vi "Reacquire Image.vi"(6 "Console Log in":refnum<class "Console Log.lvclass">, 7 "Gantry in":refnum<class "Gantry Class.lvclass">, 8 "error in":errorcluster, 9 "Tool Chuck?":T1(ring), 10 "Chuck":i32, 11 "Fiducial Image In":T3) -> (0 "error out":errorcluster, 3 "Fiducial Image Out":T3, 4 "Console Log out":refnum<class "Console Log.lvclass">, 5 "Gantry out":refnum<class "Gantry Class.lvclass">)   [LabVIEW 2011]
uses:
  Shared Components/Utils/Type Definitions/Fiducial Image.ctl
  Shared Components/Vec3d Class/Vec3d Class.lvclass
  Shared Components/Utils/Type Definitions/Physical Image.ctl
  <vilib>/vision/Image Controls.llb/IMAQ Image.ctl
  Shared Components/Utils/Type Definitions/Fiducial with Source.ctl
  Shared Components/Gantry Class/Gantry Class.lvclass
  Console Log/Console Log.lvclass
  Shared Components/Config Manager Class/Type Definitions/Named Position.ctl
  Shared Components/Config Manager Class/Type Definitions/Camera Enum.ctl
panel:
  out "Current Position":cluster{"X":dbl, "Y":dbl, "Z":dbl}
  in  "Accept":bool
  out "Preview":T2(plugin-control)
  # "Use MPG To locate fiducial\nand bring it into focus.\n\nClick \"Accept\" when\nsatisfied."
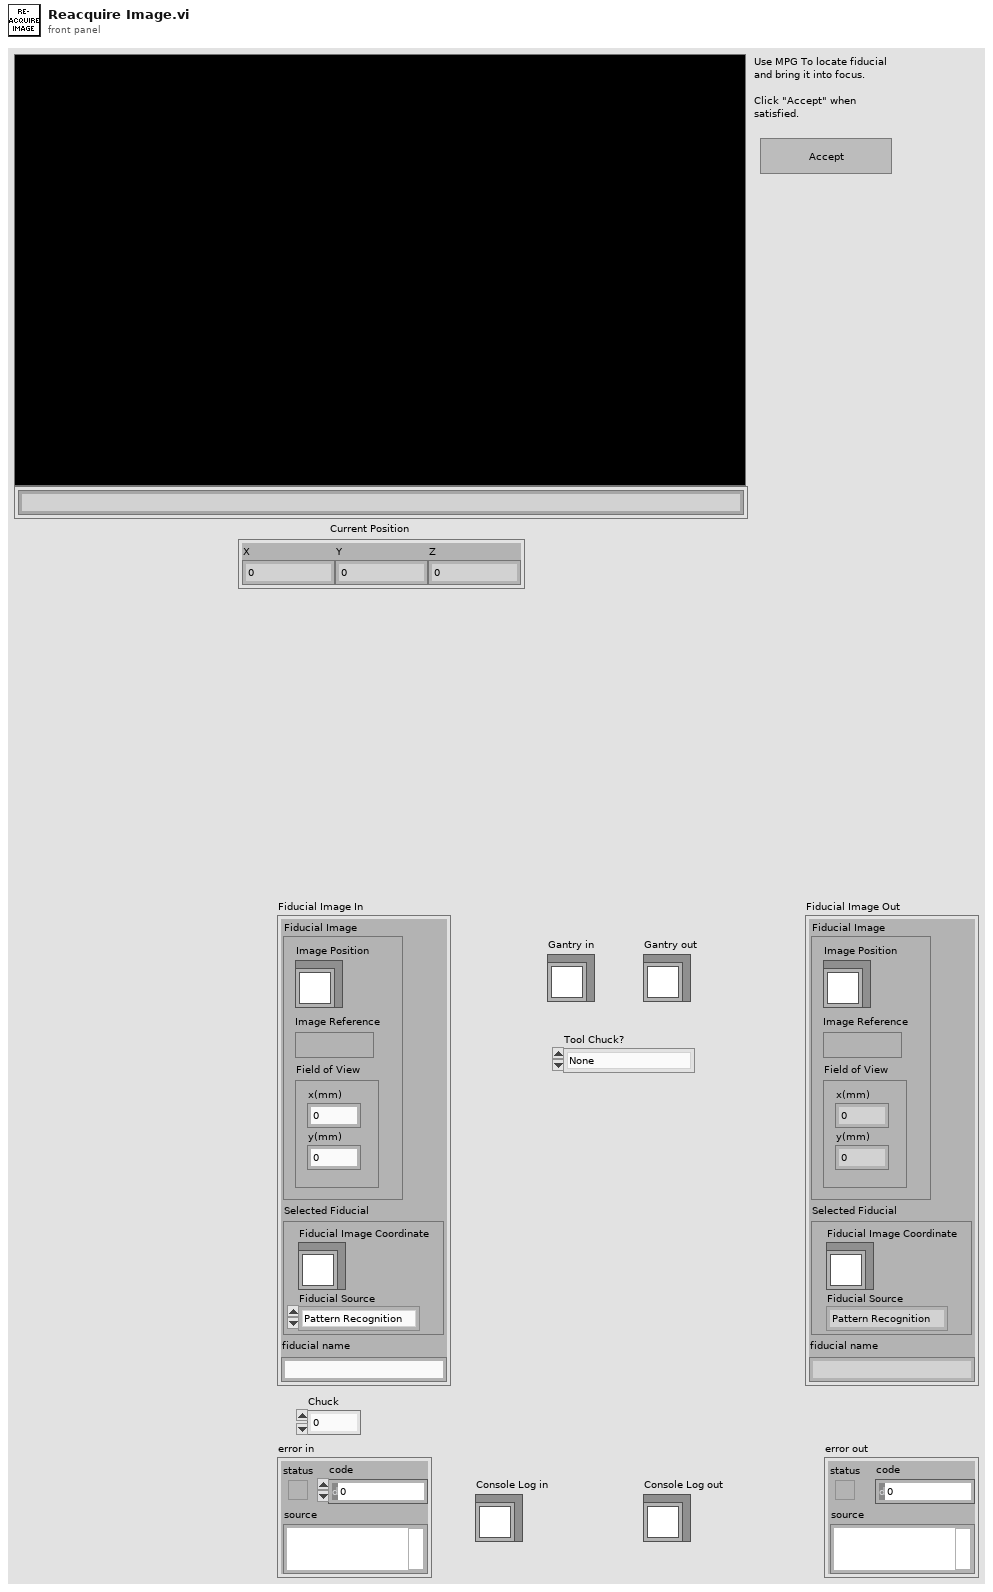
[diagram p1: front panel]
types:
  T1 = enum16{"None", "glue_resevoir_chuck", "stamp_tool_chuck", "weight_tool_chuck"}
  T2 = typedef "IMAQ Image.ctl" = refnum<image>
  T3 = typedef "Fiducial Image.ctl" = cluster{"Fiducial Image":T4, "Selected Fiducial":T5, "fiducial name":string}
  T4 = typedef "Physical Image.ctl" = cluster{"Image Position":refnum<class "Vec3d Class.lvclass">, "Image Reference":T2, "Field of View":cluster{"x(mm)":dbl, "y(mm)":dbl}}
  T5 = typedef "Fiducial with Source.ctl" = cluster{"Fiducial Image Coordinate":refnum<class "Vec3d Class.lvclass">, "Fiducial Source":enum16{"Pattern Recognition", "User", "Error", "Default"}}
  T6 = typedef "Named Position.ctl" = enum16{"home", "module_chuck_0", "module_chuck_1", "module_chuck_2", "module_chuck_3", "module_chuck_4", "glue_reservoir_chuck", "stamp_tool_chuck", "weight_tool_chuck", "needle_calibration", "tool_rack_pos_0_in", "tool_rack_pos_0_out", "tool_rack_pos_1_in", "tool_rack_pos_1_out", "tool_rack_pos_2_in", "tool_rack_pos_2_out", "front_load_position", "grabber_start_pos", "between_chuck_0_and_1", "between_chuck_2_and_3"}
  T7 = enum16{"Pattern Recognition", "User", "Error", "Default"}
  T8 = typedef "Camera Enum.ctl" = enum16{"GANTRY HEAD", "NEEDLE CALIBRATION X", "NEEDLE CALIBRATION Y"}
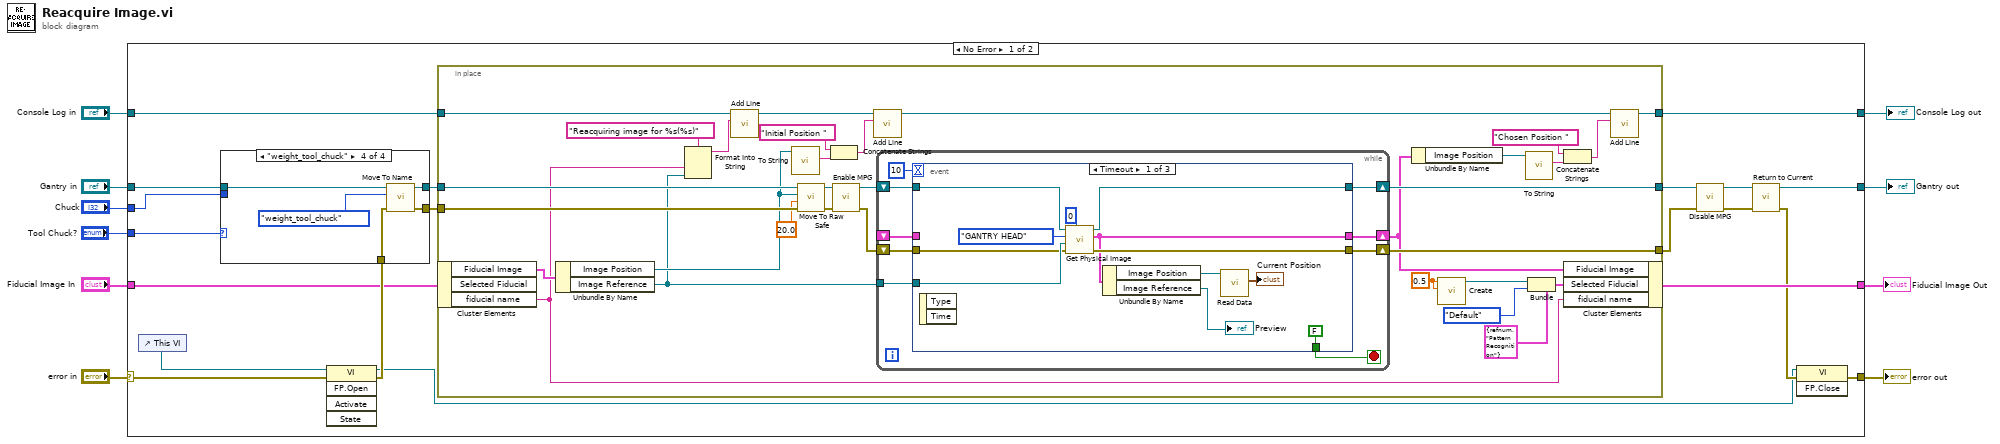
[diagram p0: block diagram]
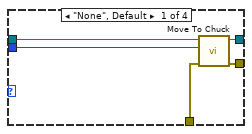
[diagram p2: hidden frame]
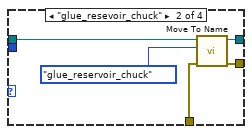
[diagram p3: hidden frame]
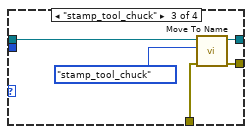
[diagram p4: hidden frame]
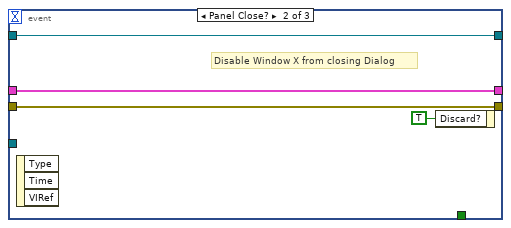
[diagram p5: hidden frame]
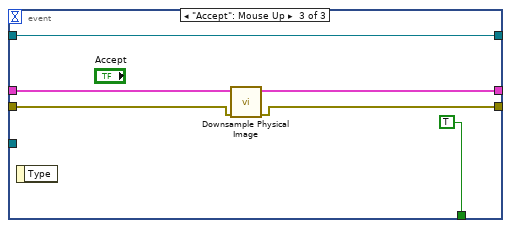
[diagram p6: hidden frame]
diagram:
  n1 = case shown="No Error" "error in" {
    selector: "error in" -> [w29 w117]
    tunnel: [w15 w117] -> w9
    tunnel: "Fiducial Image In" -> [w24 w115]
    tunnel: "Gantry in" -> [w28 w116]
    tunnel: [w18 w116] -> w6
    tunnel: "Chuck" -> [w26 _]
    tunnel: [w22 w115] -> w4
    tunnel: "Console Log in" -> [w13 w114]
    tunnel: [w12 w114] -> w2
    tunnel: "Tool Chuck?" -> [w11 _]
    frame No Error {
      n2 = control-ref of="This VI"() -> (w30:refnum<vi>)
      n3 = invoke class="VI" method="FP.Open"(reference=w30, error in=w29) -> (reference out=w14:refnum<vi>, error out=w27:errorcluster)  [unwired: 3 in, 3 out]
      n4 = case shown="\"weight_tool_chuck\"" w11 {
        tunnel: w28 -> [w35 w37 w42 w47]
        tunnel: w27 -> [w34 w38 w43 w48]
        tunnel: w26 -> [w33 _ _ _]
        tunnel: [w32 w40 w45 w50] -> w25
        tunnel: [w31 w39 w44 w49] -> w23
        frame "None", Default {
          n5 = call-dynamic "Move To Chuck.vi"("error in"=w34, "Chuck"=w33, "Gantry in"=w35) -> ("error out"=w31:errorcluster, "Gantry out"=w32:refnum<class "Gantry Class.lvclass">)  [unwired: 7 in]
        }
        frame "glue_resevoir_chuck" {
          n6 = call-dynamic "Move To Name.vi"("error in"=w38, "Destination"=Named_Position."glue_reservoir_chuck", "Gantry in"=w37) -> ("error out"=w39:errorcluster, "Gantry out"=w40:refnum<class "Gantry Class.lvclass">)  [unwired: 7 in]
        }
        frame "stamp_tool_chuck" {
          n7 = call-dynamic "Move To Name.vi"("error in"=w43, "Destination"=Named_Position."stamp_tool_chuck", "Gantry in"=w42) -> ("error out"=w44:errorcluster, "Gantry out"=w45:refnum<class "Gantry Class.lvclass">)  [unwired: 7 in]
        }
        frame "weight_tool_chuck" {
          n8 = call-dynamic "Move To Name.vi"("error in"=w48, "Destination"=Named_Position."weight_tool_chuck", "Gantry in"=w47) -> ("error out"=w49:errorcluster, "Gantry out"=w50:refnum<class "Gantry Class.lvclass">)  [unwired: 7 in]
        }
      }
      n9 = in-place {
        in-place-border: w25 -> [w82]
        in-place-border: w23 -> [w81]
        in-place-border: [w75] -> w21
        in-place-border: [w74] -> w20
        in-place-border: w13 -> [w68]
        in-place-border: [w57] -> w12
        w71 = 0.5 ("X")
        n10 = in-place-cluster #1(w24) -> ("Fiducial Image"=w76:T4, "fiducial name"=w53:string)  [unwired: 1 out]
        n11 = Unbundle By Name(w76) -> ("Image Position"=w67:refnum<class "Vec3d Class.lvclass">, "Image Reference"=w52:T2)
        n12 = Format Into String(format string="Reacquiring image for %s(%s)", w53, w52) -> (resulting string=w54:string)  [unwired: 2 in, 1 out]
        n13 = call "Add Line.vi"("String"=w54, "Console Log in"=w68) -> ("Console Log out"=w66:refnum<class "Console Log.lvclass">)  [unwired: 8 in, 1 out]
        n14 = call "To String.vi"("Vec3d in"=w67) -> ("Vec3d String"=w65:string)  [unwired: 8 in, 2 out]
        n15 = call-dynamic "Move To Raw Safe.vi"("error in"=w81, "Speed(mm/s)"=20.0, "Destination"=w67, "Gantry in"=w82) -> ("error out"=w78:errorcluster, "Gantry out"=w80:refnum<class "Gantry Class.lvclass">)  [unwired: 6 in]
        n16 = Concatenate Strings("Initial Position ", w65) -> (w63:string)
        n17 = call-dynamic "Enable MPG.vi"("error in"=w78, "Gantry in"=w80) -> ("error out"=w77:errorcluster, "Gantry out"=w79:refnum<class "Gantry Class.lvclass">)  [unwired: 8 in]
        n18 = call "Add Line.vi"("String"=w63, "Console Log in"=w66) -> ("Console Log out"=w58:refnum<class "Console Log.lvclass">)  [unwired: 8 in, 1 out]
        n19 = while {
          tunnel: w52 -> [w88]
          shift-right: [w85] -> w75
          shift-left: w79 -> [w89]
          shift-right: [w84] -> w60
          shift-left: _ -> [w83]
          shift-right: [w86] -> w74
          shift-left: w77 -> [w87]
          stop <- w90 stop-if-true
          n20 = event shown="[0] Timeout" {
            selector: _ -> [_ _ _]
            dyn-events: _ -> [_ _ _]
            timeout: 10 -> [_ _ _]
            tunnel: [FALSE _ TRUE] -> w90
            tunnel: w89 -> [w102 w106 w112]
            tunnel: w88 -> [w99 _ _]
            tunnel: w87 -> [w98 w104 w109]
            tunnel: [w94 w104 w108] -> w86
            tunnel: [w93 w106 w112] -> w85
            tunnel: [w92 w105 w110] -> w84
            tunnel: w83 -> [_ w105 w111]
            event Timeout {
              n21 = event-data() -> ()  [unwired: 1 in, 2 out]
              n22 = call-dynamic "Get Physical Image.vi"("Delay(milliseconds)"=0, "error in"=w98, "Image In"=w99, "Camera Name"=Camera_Enum."GANTRY HEAD", "Gantry in"=w102) -> ("error out"=w94:errorcluster, "Physical Image"=w92:T4, "Gantry out"=w93:refnum<class "Gantry Class.lvclass">)  [unwired: 4 in]
              n23 = Unbundle By Name(w92) -> ("Image Position"=w96:refnum<class "Vec3d Class.lvclass">, "Image Reference"=→"Preview":T2)
              n24 = call-dynamic "Read Data.vi"("Vec3d Class in"=w96) -> ("Data"=→"Current Position":cluster{"X":dbl, "Y":dbl, "Z":dbl})  [unwired: 8 in, 2 out]
            }
            event Panel Close? {
              # "Disable Window X from closing Dialog"
              n25 = event-data() -> ()  [unwired: 1 in, 3 out]
              n26 = event-data("Discard?"=TRUE) -> ()  [unwired: 1 in, 1 out]
            }
            event "Accept": Mouse Up {
              n27 = event-data() -> ()  [unwired: 1 in, 1 out]
              n28 = call "Downsample Physical Image.vi"("error in"=w109, "Physical Image In"=w111) -> ("error out"=w108:errorcluster, "Physical Image Out"=w110:T4)  [unwired: 8 in]
            }
          }
        }
        n29 = Unbundle By Name(w60) -> ("Image Position"=w59:refnum<class "Vec3d Class.lvclass">)
        n30 = call "Create.vi"("Y"=w71, "X"=w71) -> ("Vec3d Class out"=w72:refnum<class "Vec3d Class.lvclass">)  [unwired: 8 in, 1 out]
        n31 = call "To String.vi"("Vec3d in"=w59) -> ("Vec3d String"=w62:string)  [unwired: 8 in, 2 out]
        n32 = Bundle(cluster=T5 {"Fiducial Image Coordinate"=refnum, "Fiducial Source"=enum."Pattern Recognition"} ("Selected Fiducial"), "Fiducial Image Coordinate"=w72, "Fiducial Source"=T7."Default") -> (w69:T5)
        n33 = Concatenate Strings("Chosen Position ", w62) -> (w56:string)
        n34 = in-place-cluster #1("Fiducial Image"=w60, "Selected Fiducial"=w69, "fiducial name"=w53) -> (w22:T3)
        n35 = call "Add Line.vi"("String"=w56, "Console Log in"=w58) -> ("Console Log out"=w57:refnum<class "Console Log.lvclass">)  [unwired: 8 in, 1 out]
      }
      n36 = call-dynamic "Disable MPG.vi"("error in"=w20, "Gantry in"=w21) -> ("error out"=w17:errorcluster, "Gantry out"=w19:refnum<class "Gantry Class.lvclass">)  [unwired: 8 in]
      n37 = call-dynamic "Return to Current.vi"("error in"=w17, "Gantry in"=w19) -> ("error out"=w16:errorcluster, "Gantry out"=w18:refnum<class "Gantry Class.lvclass">)  [unwired: 8 in]
      n38 = invoke class="VI" method="FP.Close"(reference=w14, error in=w16) -> (error out=w15:errorcluster)  [unwired: 1 in, 2 out]
    }
    frame Error {
    }
  }
  "Fiducial Image Out" <- w4
  "error out" <- w9
  "Gantry out" <- w6
  "Console Log out" <- w2
